vi "AO_Loop.vi"(8 "error":errorcluster) -> (0 "error out":errorcluster)   [LabVIEW 2018]
doc: "This example demonstrates how to generate a user-defined voltage using the analog output of a DAQ device."
uses:
  Controls/Enums/AO_Loop_Enum.ctl
  <vilib>/DAQmx/write.llb/DAQmx Write (Analog 1D DBL NChan 1Samp).vi
  <vilib>/DAQmx/create/channels.llb/DAQmx Create Channel (AO-Voltage-Basic).vi
  <vilib>/DAQmx/miscellaneous.llb/DAQmx Fill In Error Info.vi
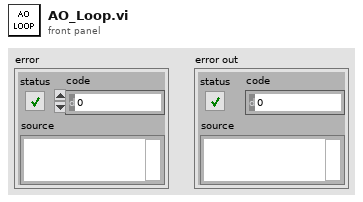
[diagram p1: front panel]
types:
  T1 = typedef "AO_Loop_Enum.ctl" = enum16{"AO_Init", "AO_Write", "AO_Exit"}
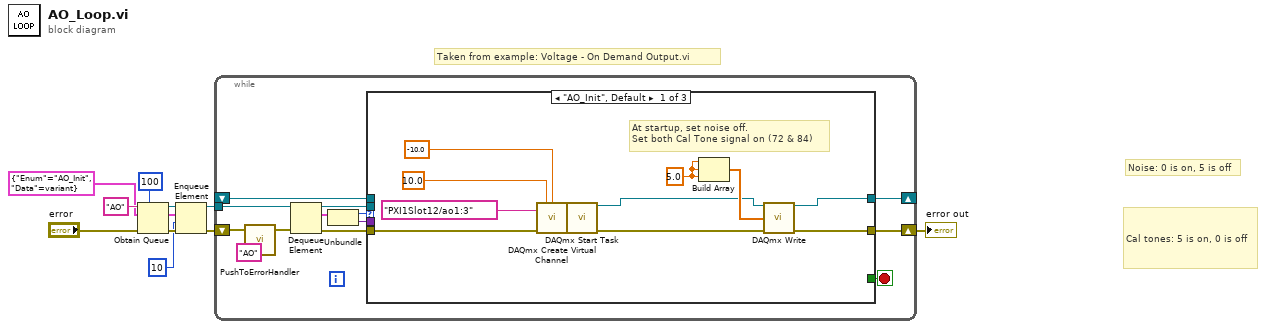
[diagram p0: block diagram]
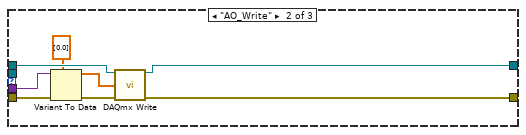
[diagram p2: hidden frame]
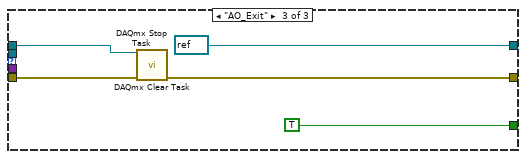
[diagram p3: hidden frame]
diagram:
  w6 = cluster{"Enum":T1, "Data":variant} {"Enum"=enum."AO_Init", "Data"=variant}
  # "Cal tones: 5 is on, 0 is off"
  # "Noise: 0 is on, 5 is off"
  # "Taken from example: Voltage - On Demand Output.vi"
  n1 = Obtain Queue(max queue size (-1, unlimited)=100, name (unnamed)="AO", element data type=w6, error in (no error)="error") -> (queue out=w10:refnum<queue>, error out=w8:errorcluster)  [unwired: 1 in, 1 out]
  n2 = Enqueue Element(queue=w10, element=w6, timeout in ms (-1)=10, error in (no error)=w8) -> (queue out=w9:refnum<queue>, error out=w2:errorcluster)  [unwired: 1 out]
  n3 = while {
    tunnel: w9 -> [w20]
    shift-right: [w22] -> w4
    shift-left: w2 -> [w12]
    shift-right: [w23] -> _
    shift-left: _ -> [w16]
    stop <- w14 stop-if-true
    n4 = call "PushToErrorHandler.vi"("ErrorIn"=w12, "ErrorLocation"="AO") -> ("ErrorOut"=w13:errorcluster)  [unwired: 5 in]
    n5 = Dequeue Element(queue=w20, error in (no error)=w13) -> (queue out=w15:refnum<queue>, element=w19:cluster{"Enum":T1, "Data":variant}, error out=w21:errorcluster)  [unwired: 1 in, 1 out]
    n6 = Unbundle(w19) -> ("Enum"=w18:T1, "Data"=w17:variant)
    n7 = case shown="\"AO_Init\", Default" w18 {
      tunnel: w16 -> [_ w43 w46]
      tunnel: w21 -> [w30 w40 w48]
      tunnel: [w24 w42 refnum<k21> refnum ("task out")] -> w23
      tunnel: [w27 w41 w47] -> w22
      tunnel: w17 -> [_ w38 _]
      tunnel: w15 -> [_ _ _]
      tunnel: [_ _ TRUE] -> w14
      frame "AO_Init", Default {
        w29 = 5.0
        # "At startup, set noise off.\nSet both Cal Tone signal on (72 & 84)"
        n8 = call-poly <vilib>:"DAQmx Create Virtual Channel.vi"("maximum value"=10.0 ("Max Voltage"), "minimum value"=-10.0 ("Min Voltage"), "physical channels"=tag "PXI1Slot12/ao1:3" ("Physical Channel(s)"), "error in"=w30) -> ("task out"=w34:refnum<k21>, "error out"=w35:errorcluster)  [unwired: 10 in]
        n9 = call <vilib>:"DAQmx Start Task.vi"("task/channels in"=w34, "error in"=w35) -> ("task out"=w25:refnum<k21>, "error out"=w28:errorcluster)  [unwired: 12 in]
        n10 = Build Array(w29, w29, w29) -> (w26:dbl[])
        n11 = call-poly <vilib>:"DAQmx Write.vi"("task/channels in"=w25, "data"=w26, "error in"=w28) -> ("task out"=w24:refnum<k21>, "error out"=w27:errorcluster)  [unwired: 10 in, 1 out]
      }
      frame "AO_Write" {
        n12 = Variant To Data(error in=w40, type=dbl[] [0.0] ("Output Array"), Variant=w38) -> (data=w36:dbl[], error out=w39:errorcluster)
        n13 = call-poly <vilib>:"DAQmx Write.vi"("task/channels in"=w43, "data"=w36, "error in"=w39) -> ("task out"=w42:refnum<k21>, "error out"=w41:errorcluster)  [unwired: 10 in, 1 out]
      }
      frame "AO_Exit" {
        n14 = call <vilib>:"DAQmx Stop Task.vi"("task/channels in"=w46, "error in"=w48) -> ("task out"=w49:refnum<k21>, "error out"=w50:errorcluster)  [unwired: 12 in]
        n15 = call <vilib>:"DAQmx Clear Task.vi"("task in"=w49, "error in"=w50) -> ("error out"=w47:errorcluster)  [unwired: 13 in]
      }
    }
  }
  "error out" <- w4
